vi "api_mqttConnect.vi"(11 "error in (no error)":errorcluster) -> (4 "success":bool, 6 "connStatus":T1=enum."Connection refused: not authorized", 8 "sessionPresent":bool, 15 "error out":errorcluster)   [LabVIEW 2021, in "mqtt.lvclass"]
uses:
  mqtt.lvclass
  mqttTypedef/mqttConnectionStatus.ctl
  mqttCmd/mqttCmdConnect/mqttCmdConnect.lvclass
  C:/Users/Fujitsu/Desktop/labpublish/avril/Project mqtt/Src/class/mqtt/mqttCmd/mqttCmd.lvclass
  mqttTypedef/mqttQOSlevel.ctl
  mqttConfigFunction.ctl
  mqttTypedef/mqttMessageType.ctl
  mqttCmd/mqttCmdConnect/mqttCmdConnect.lvclass/mqttCmdConnect.ctl
  mqttCmd/mqttCmd.lvclass/mqttCmd.ctl
  mqttCmd/mqttCmd.lvclass
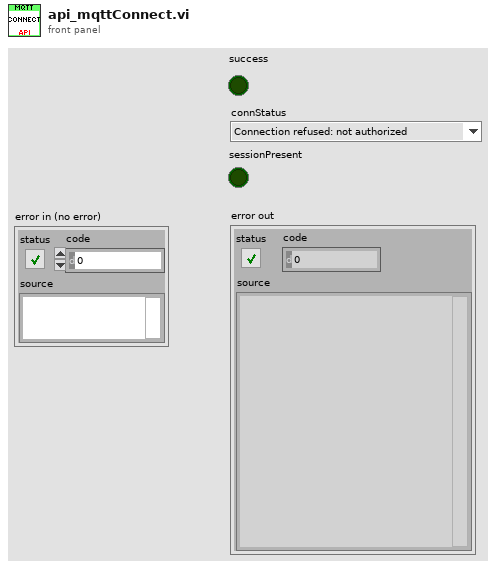
[diagram p1: front panel]
types:
  T1 = typedef "mqttConnectionStatus.ctl" = enum16{"Connection accepted", "Connection refused: unacceptable protocol version", "Connection refused: identifier rejected", "Connection refused: Server unavailable", "Connection refused: bad user name or password", "Connection refused: not authorized"}
  T2 = typedef "mqttMessageType.ctl" = enum32{"Reserved", "CONNECT", "CONNACK", "PUBLISH", "PUBACK", "PUBREC", "PUBREL", "PUBCOMP", "SUBSCRIBE", "SUBACK", "UNSUBSCRIBE", "UNSUBACK", "PINGREQ", "PINGRESP", "DISCONNECT", "Reserved2"}
  T3 = typedef "mqtt.lvclass/mqttConfigFunction.ctl" = enum16{"init", "deinit", "set", "get"}
  T4 = typedef "mqttQOSlevel.ctl" = enum8{"At most once", "At least once", "Exactly once", "Reserved"}
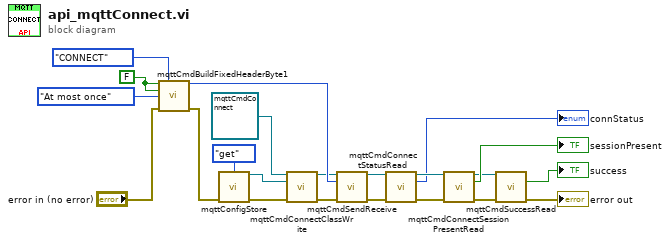
[diagram p0: block diagram]
diagram:
  w19 = FALSE
  n1 = call "mqttCmdBuildFixedHeaderByte1.vi"("retain(F)"=w19, "MessageType"=mqttMessageType."CONNECT", "duplicate(F)"=w19, "QoS (At most once)"=mqttQOSlevel."At most once", "error in (no error)"="error in (no error)") -> ("byte1"=w21:u8, "error out"=w16:errorcluster)  [unwired: 9 in]
  n2 = call "mqttConfigStore.vi"("function"=mqttConfigFunction."get", "error in (no error)"=w16) -> ("mqtt.lvclass out"=w14:refnum<class "mqtt.lvclass">, "error out"=w15:errorcluster)  [unwired: 12 in]
  n3 = call "mqttCmdConnectClassWrite.vi"("mqttConnect in"=refnum<class "mqttCmdConnect.lvclass"> refnum ("mqttConnect.lvclass"), "mqtt.lvclass"=w14, "error in (no error)"=w15) -> ("mqttConnect out"=w12:refnum<class "mqttCmdConnect.lvclass">, "error out"=w11:errorcluster)  [unwired: 11 in]
  n4 = call "mqttCmdSendReceive.vi"("mqttConnect in"=w12, "byte1"=w21, "error in (no error)"=w11) -> ("mqttConnect out"=w2:refnum<class "mqttCmdConnect.lvclass">, "error out"=w1:errorcluster)  [unwired: 10 in, 1 out]
  n5 = call "mqttCmdConnectStatusRead.vi"("mqttConnect in"=w2, "error in (no error)"=w1) -> ("mqttConnect out"=w9:refnum<class "mqttCmdConnect.lvclass">, "connStatus"=→"connStatus":T1, "error out"=w10:errorcluster)  [unwired: 11 in]
  n6 = call "mqttCmdConnectSessionPresentRead.vi"("mqttConnect in"=w9, "error in (no error)"=w10) -> ("mqttConnect out"=w4:refnum<class "mqttCmdConnect.lvclass">, "sessionPresent"=→"sessionPresent":bool, "error out"=w6:errorcluster)  [unwired: 11 in]
  n7 = call "mqttCmdSuccessRead.vi"("mqttBrokerCommand in"=w4, "error in (no error)"=w6) -> ("success"=→"success":bool, "error out"=→"error out":errorcluster)  [unwired: 11 in, 1 out]
